vi "Reinitialize.vi"(8 "error in (no error)":errorcluster, 11 "TroSpec in":refnum<class "PL ISTEQ TroSpec.lvclass">) -> (0 "error out":errorcluster, 3 "TroSpec out":refnum<class "PL ISTEQ TroSpec.lvclass">)   [LabVIEW 2015, in "PL ISTEQ TroSpec.lvclass"]
doc: "Reinitializes connection to device based on previously specified settings."
uses:
  PL ISTEQ TroSpec.lvclass
  PL ISTEQ TroSpec.lvclass/PL ISTEQ TroSpec.ctl
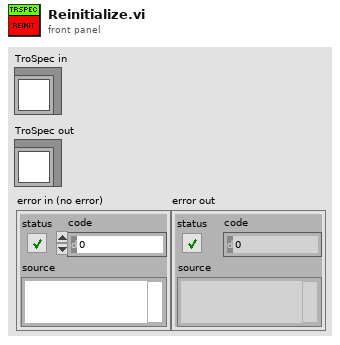
[diagram p1: front panel]
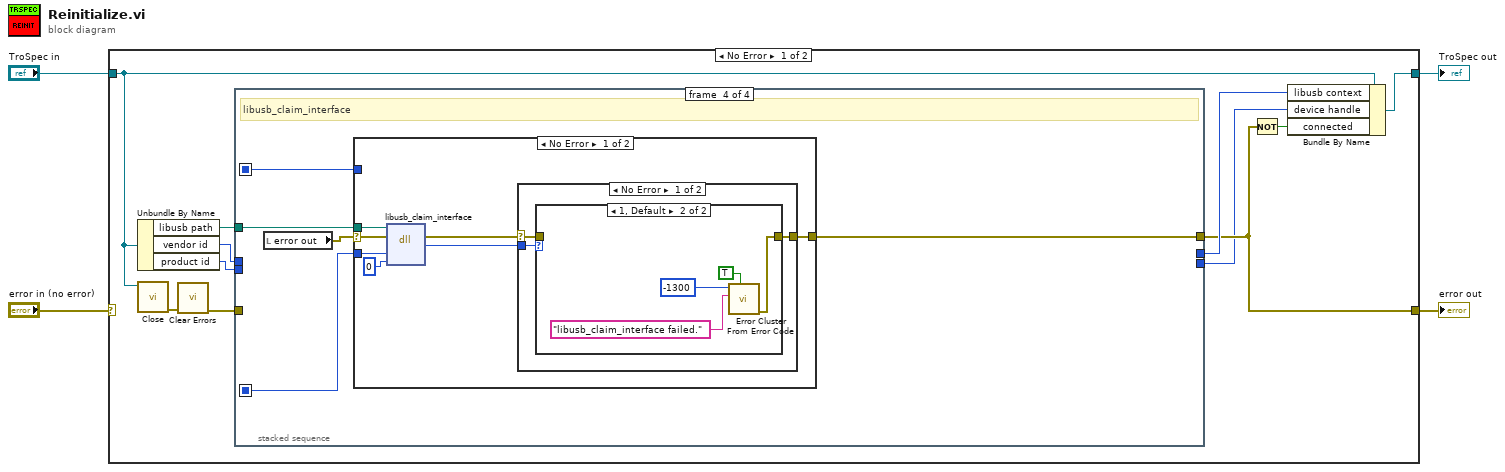
[diagram p0: block diagram]
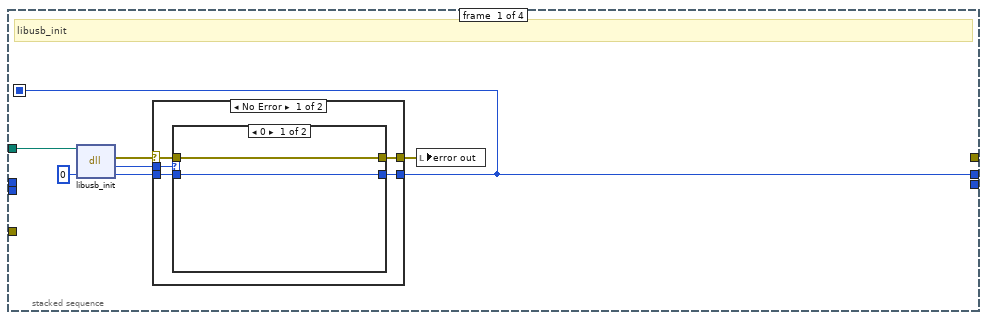
[diagram p2: hidden frame]
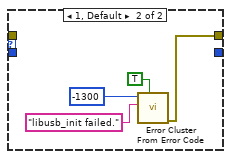
[diagram p3: hidden frame]
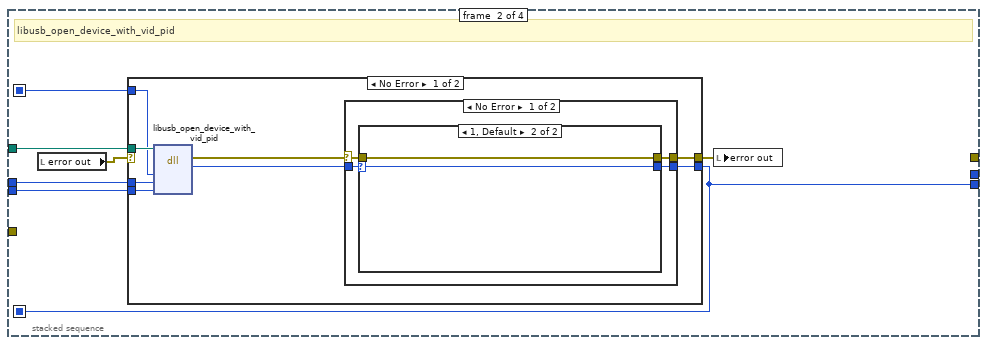
[diagram p5: hidden frame]
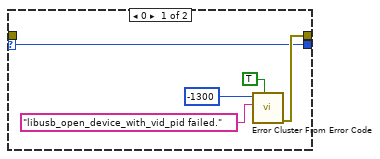
[diagram p6: hidden frame]
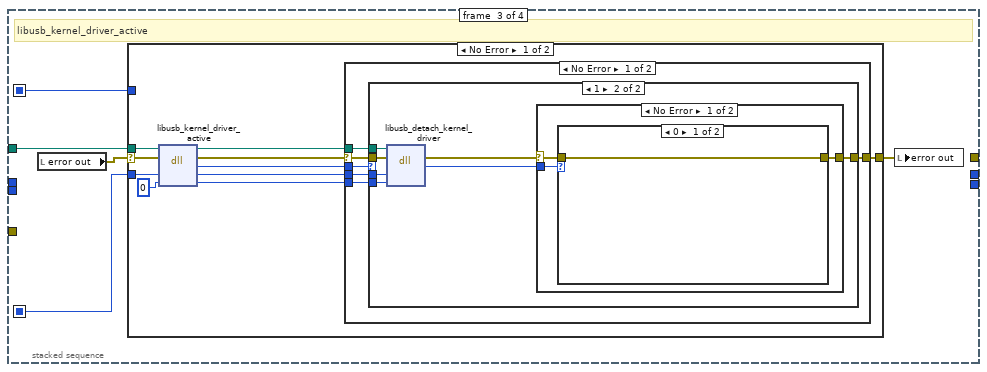
[diagram p9: hidden frame]
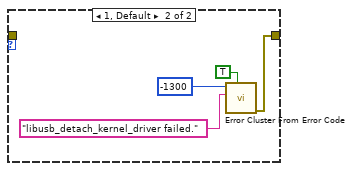
[diagram p11: hidden frame]
diagram:
  n1 = case shown="No Error" "error in (no error)" {
    selector: "error in (no error)" -> [_ w126]
    tunnel: [w6 w126] -> w4
    tunnel: "TroSpec in" -> [w13 w125]
    tunnel: [w14 w125] -> w1
    frame No Error {
      n2 = Unbundle By Name(w13) -> ("libusb path"=w11:path, "vendor id"=w8:u16, "product id"=w7:u16)
      n3 = call "Close.vi"("TroSpec in"=w13) -> ("error out"=w15:errorcluster)  [unwired: 10 in]
      n4 = call <vilib>:"Clear Errors.vi"("error in (no error)"=w15) -> ("error out"=w10:errorcluster)  [unwired: 5 in, 1 out]
      n5 = stacked-sequence {
        seq-local: [w16 _ _ _] -> [_ w39 w65 w105]
        seq-local: [_ w37 _ _] -> [_ _ w63 w104]
        tunnel: w11 -> [w21 w40 w66 w106]
        tunnel: w10 -> [_ _ _ _]
        tunnel: [w16 _ _ _] -> w9
        tunnel: [_ w37 _ _] -> w5
        tunnel: w8 -> [_ w36 _ _]
        tunnel: w7 -> [_ w35 _ _]
        tunnel: [_ _ _ w103] -> w6
        frame #0 {
          # "libusb_init"
          n6 = dll-call lib="D:/GitHub/temp/isteq-trospec-labview/Public/libusb-1.0-x64.dll" fn="libusb_init"(path in=w21, "ctx"=u64 0) -> (error out=w20:errorcluster, "return type"=w18:i32, "ctx"=w19:u64)  [unwired: 2 in, 1 out]
          n7 = case shown="No Error" w20 {
            selector: w20 -> [w24 w34]
            tunnel: w19 -> [w26 _]
            tunnel: w18 -> [w27 _]
            tunnel: [w25 w34] -> w17
            tunnel: [w23 _] -> w16
            frame No Error {
              n8 = case shown="0" w27 {
                tunnel: w26 -> [w28 _]
                tunnel: [w29 w30] -> w25
                tunnel: w24 -> [w29 _]
                tunnel: [w28 _] -> w23
                frame 0 {
                }
                frame 1, Default {
                  n9 = call <vilib>:"Error Cluster From Error Code.vi"("show call chain? (False)"=TRUE, "error message (\"\")"="libusb_init failed." ("format string"), "error code (0)"=-1300) -> ("error out"=w30:errorcluster)  [unwired: 6 in]
                }
              }
            }
            frame Error {
            }
          }
          n10 = local write "error out"(w17) -> ()
        }
        frame #1 {
          # "libusb_open_device_with_vid_pid"
          n11 = local read "error out"() -> (w41:errorcluster)
          n12 = case shown="No Error" w41 {
            selector: w41 -> [_ w62]
            tunnel: w40 -> [w49 _]
            tunnel: [w44 w62] -> w38
            tunnel: w39 -> [w48 _]
            tunnel: [w45 _] -> w37
            tunnel: w36 -> [w43 _]
            tunnel: w35 -> [w42 _]
            frame No Error {
              n13 = dll-call lib="D:/GitHub/temp/isteq-trospec-labview/Public/libusb-1.0-x64.dll" fn="libusb_open_device_with_vid_pid"(path in=w49, "ctx"=w48, "vendor_id"=w43, "product_id"=w42) -> (error out=w47:errorcluster, "return type"=w46:u64)  [unwired: 5 in, 1 out]
              n14 = case shown="No Error" w47 {
                selector: w47 -> [w51 w61]
                tunnel: w46 -> [w53 _]
                tunnel: [w52 w61] -> w44
                tunnel: [w50 _] -> w45
                frame No Error {
                  n15 = case shown="1, Default" w53 {
                    selector: w53 -> [w54 w59]
                    tunnel: [w55 w60] -> w52
                    tunnel: w51 -> [_ w60]
                    tunnel: [w54 w59] -> w50
                    frame 0 {
                      n16 = call <vilib>:"Error Cluster From Error Code.vi"("show call chain? (False)"=TRUE, "error message (\"\")"="libusb_open_device_with_vid_pid failed." ("format string"), "error code (0)"=-1300) -> ("error out"=w55:errorcluster)  [unwired: 6 in]
                    }
                    frame 1, Default {
                    }
                  }
                }
                frame Error {
                }
              }
            }
            frame Error {
            }
          }
          n17 = local write "error out"(w38) -> ()
        }
        frame #2 {
          # "libusb_kernel_driver_active"
          n18 = local read "error out"() -> (w67:errorcluster)
          n19 = case shown="No Error" w67 {
            selector: w67 -> [w75 w102]
            tunnel: w66 -> [w76 _]
            tunnel: [w77 w102] -> w64
            tunnel: w65 -> [_ _]
            tunnel: w63 -> [w73 _]
            frame No Error {
              n20 = dll-call lib="D:/Temp/libusb/libusb-1.0-x64.dll" fn="libusb_kernel_driver_active"(path in=w76, error in=w75, "dev_handle"=w73, "interface_number"=0) -> (path out=w68:path, error out=w74:errorcluster, "return type"=w70:i32, "dev_handle"=w71:u64, "interface_number"=w69:i32)  [unwired: 1 in]
              n21 = case shown="No Error" w74 {
                selector: w74 -> [w83 w101]
                tunnel: [w78 w101] -> w77
                tunnel: w71 -> [w81 _]
                tunnel: w70 -> [w79 _]
                tunnel: w69 -> [w80 _]
                tunnel: w68 -> [w82 _]
                frame No Error {
                  n22 = case shown="1" w79 {
                    tunnel: w83 -> [w84 w91]
                    tunnel: w81 -> [_ w90]
                    tunnel: w82 -> [_ w89]
                    tunnel: w80 -> [_ w88]
                    tunnel: [w84 w85] -> w78
                    frame 0, Default {
                    }
                    frame 1 {
                      n23 = dll-call lib="D:/Temp/libusb/libusb-1.0-x64.dll" fn="libusb_detach_kernel_driver"(path in=w89, error in=w91, "dev_handle"=w90, "interface_number"=w88) -> (error out=w87:errorcluster, "return type"=w86:i32)  [unwired: 3 in, 1 out]
                      n24 = case shown="No Error" w87 {
                        selector: w87 -> [w93 w100]
                        tunnel: w86 -> [w94 _]
                        tunnel: [w92 w100] -> w85
                        frame No Error {
                          n25 = case shown="0" w94 {
                            tunnel: w93 -> [w95 _]
                            tunnel: [w95 w97] -> w92
                            frame 0 {
                            }
                            frame 1, Default {
                              n26 = call <vilib>:"Error Cluster From Error Code.vi"("show call chain? (False)"=TRUE, "error message (\"\")"="libusb_detach_kernel_driver failed." ("format string"), "error code (0)"=-1300) -> ("error out"=w97:errorcluster)  [unwired: 6 in]
                            }
                          }
                        }
                        frame Error {
                        }
                      }
                    }
                  }
                }
                frame Error {
                }
              }
            }
            frame Error {
            }
          }
          n27 = local write "error out"(w64) -> ()
        }
        frame #3 {
          # "libusb_claim_interface"
          n28 = local read "error out"() -> (w107:errorcluster)
          n29 = case shown="No Error" w107 {
            selector: w107 -> [w112 w124]
            tunnel: w106 -> [w113 _]
            tunnel: [w114 w124] -> w103
            tunnel: w105 -> [_ _]
            tunnel: w104 -> [w111 _]
            frame No Error {
              n30 = dll-call lib="D:/Temp/libusb/libusb-1.0-x64.dll" fn="libusb_claim_interface"(path in=w113, error in=w112, "dev_handle"=w111, "interface_number"=0) -> (error out=w109:errorcluster, "return type"=w108:i32)  [unwired: 3 in, 1 out]
              n31 = case shown="No Error" w109 {
                selector: w109 -> [w116 w123]
                tunnel: w108 -> [w117 _]
                tunnel: [w115 w123] -> w114
                frame No Error {
                  n32 = case shown="1, Default" w117 {
                    tunnel: w116 -> [w118 _]
                    tunnel: [w118 w120] -> w115
                    frame 0 {
                    }
                    frame 1, Default {
                      n33 = call <vilib>:"Error Cluster From Error Code.vi"("show call chain? (False)"=TRUE, "error message (\"\")"="libusb_claim_interface failed." ("format string"), "error code (0)"=-1300) -> ("error out"=w120:errorcluster)  [unwired: 6 in]
                    }
                  }
                }
                frame Error {
                }
              }
            }
            frame Error {
            }
          }
        }
      }
      n34 = Not(x=w6) -> (.not. x?=w12:bool)
      n35 = Bundle By Name(cluster=w13, "libusb context"=w9, "device handle"=w5, "connected"=w12) -> (w14:refnum<class "PL ISTEQ TroSpec.lvclass">)
    }
    frame Error {
    }
  }
  "error out" <- w4
  "TroSpec out" <- w1
